vi "Alarm Tag Generation.vi"(1 "Spreadsheet Input":string, 2 "Alarm Type":string) -> (0 "Group & CVT Tag List":cluster{string[], T1[]})   [LabVIEW 2013]
uses:
  <vilib>/NI/Current Value Table/Type Defs/Single Tag.ctl
  <vilib>/NI/Current Value Table/Type Defs/Data Types.ctl
  <vilib>/NI/Current Value Table/Current Value Table.lvlib
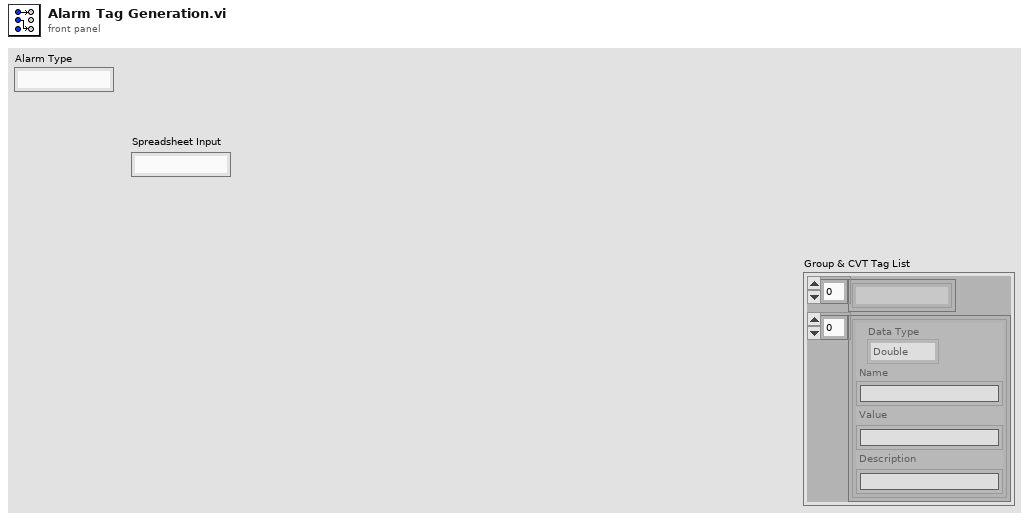
[diagram p1: front panel]
types:
  T1 = typedef "Current Value Table.lvlib/Single Tag.ctl" = cluster{"Data Type":T2, "Name":string, "Value":string, "Description":string}
  T2 = typedef "Current Value Table.lvlib/Data Types.ctl" = enum16{"Double", "Single", "I64", "I32", "I16", "I8", "U64", "U32", "U16", "U8", "String", "Boolean", "Array of U8", "Array of U16", "Array of U32", "Array of U64", "Array of I64", "Array of I32", "Array of I16", "Array of I8", "Array of Double", "Array of Single", "Array of Boolean", "Array of String"}
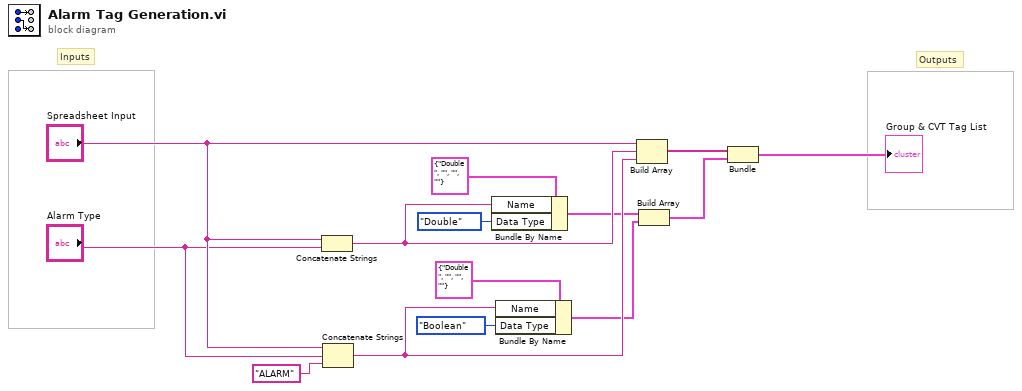
[diagram p0: block diagram]
diagram:
  # "Outputs"
  # "Inputs"
  n1 = Concatenate Strings("Spreadsheet Input", "Alarm Type") -> (w10:string)
  n2 = Concatenate Strings("Spreadsheet Input", "Alarm Type", "ALARM" ("string")) -> (w9:string)
  n3 = Bundle By Name(cluster=T1 {"Data Type"=enum."Double", "Name"="", "Value"="", "Description"=""} ("Tag"), "Name"=w10, "Data Type"=Data_Types."Double") -> (w7:T1)
  n4 = Bundle By Name(cluster=T1 {"Data Type"=enum."Double", "Name"="", "Value"="", "Description"=""} ("Tag"), "Name"=w9, "Data Type"=Data_Types."Boolean") -> (w6:T1)
  n5 = Build Array("Spreadsheet Input", w10, w9) -> (w3:string[])
  n6 = Build Array(w7, w6) -> (w2:T1[])
  n7 = Bundle(w3, w2) -> (→"Group & CVT Tag List":cluster{string[], T1[]})  [unwired: 1 in]
